vi "simulation_globals.vi"() -> ()   [LabVIEW 2010]
panel:
  out "Particle Positions":cluster{dbl, dbl, dbl}[](array[cluster])
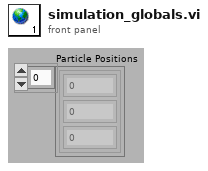
[diagram p1: front panel]
diagram:
